vi "Store_single_subvi.vi"(3 "Parameter":u32(ring)=2049184 items=["SENSOR MODE"=4212128, "CCD MODE"=4212384, "READOUT MODE"=4211872, "ACTIVE VIEW INDEX"=4343136, "BITS PER CHANNEL"=4342976, "IMAGE PIXEL TYPE"=4343296, "BINNING"=4215968, "EXPOSURE TIME"=2049184, "CONTRAST GAIN"=3163312, "CONTRAST OFFSET"=3163328, "LIGHT MODE"=2114720, "SENSITIVITY"=2114992, "PHOTON IMAGING MODE"=2115200, "HIGH DYNAMIC RANGE MODE"=3163360, "WHITE BALANCE"=3163568, "TEMPERATURE"=2115232, "TEMPERATURE TARGET"=2115264, "SENSOR COOLER FAN"=2115296, "LINEBUNDLE HEIGHT"=4212192, "MECHANICAL SHUTTER"=2115488, "BACK FOCUS POSITION"=8422304, "TRIGGER CONNECTOR"=1066432, "TRIGGER SOURCE"=1066144, "OUTPUT TRIGGER SOURCE"=1852576, "TRIGGER GLOBAL EXPOSURE"=2049680, "FIRST TRIGGER BEHAVIOR"=2049696, "CHANNEL SYNC"=1852352, "READOUT DIRECTION"=4211904, "PRE HSYNC COUNT"=1852704, "INTERNAL LINE SPEED"=4226000, "INTERNAL LINE INTERVAL"=4226016], 4 "Set":dbl=0.5, 5 "Frames":i32=1, 6 "File":path=path "D:/test", 7 "save":bool=TRUE caption="Blank Button") -> (0 "Display":T1(plugin-control), 1 "DCAM Version":string, 2 "Library Version":string)   [LabVIEW 2016]
uses:
  Global_Variates.vi
panel:
  in  "w2 2":i32
  in  "w1 2":i32
  in  "h2 2":i32
  in  "h1 2":i32
  in  "w2":i32=2048 min=0 max=2048 step=1
  in  "w1":i32 min=0 max=2048 step=1
  in  "h2":i32=2048 min=0 max=2048 step=1
  in  "h1":i32 min=0 max=2048 step=1
  out "w2-1":dbl format="%#_13g"
  out "h2-1":dbl format="%#_13g"
  # "中间亮斑"
  # "裁剪图片"
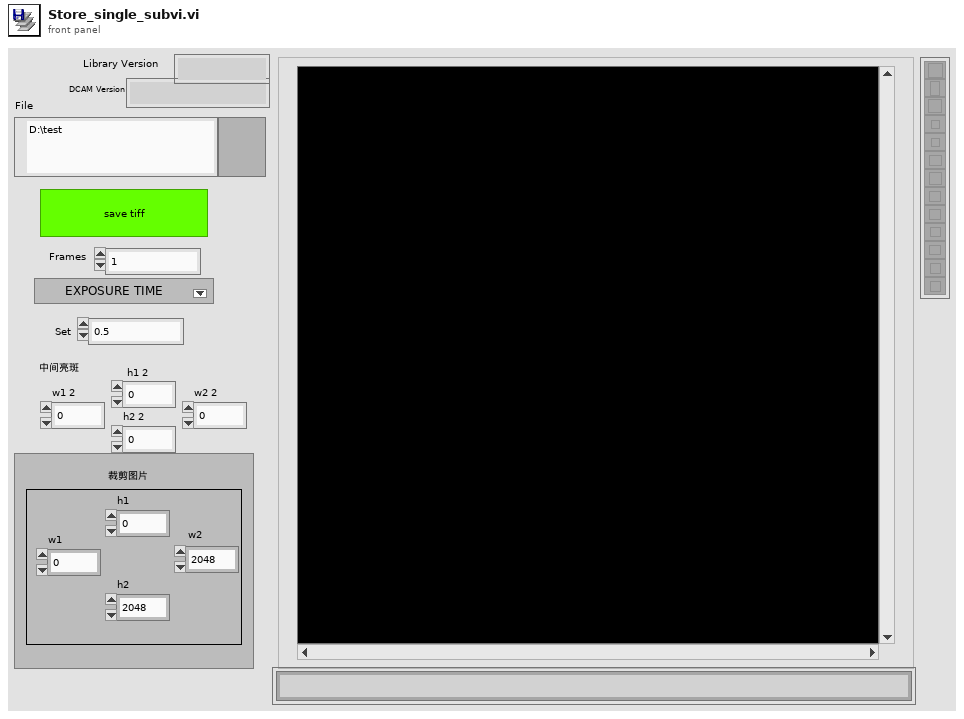
[diagram p1: front panel]
types:
  T1 = typedef "IMAQ Image.ctl" = refnum<image>
  T2 = cluster{"Capture Library":string, "DCAM-API":string}
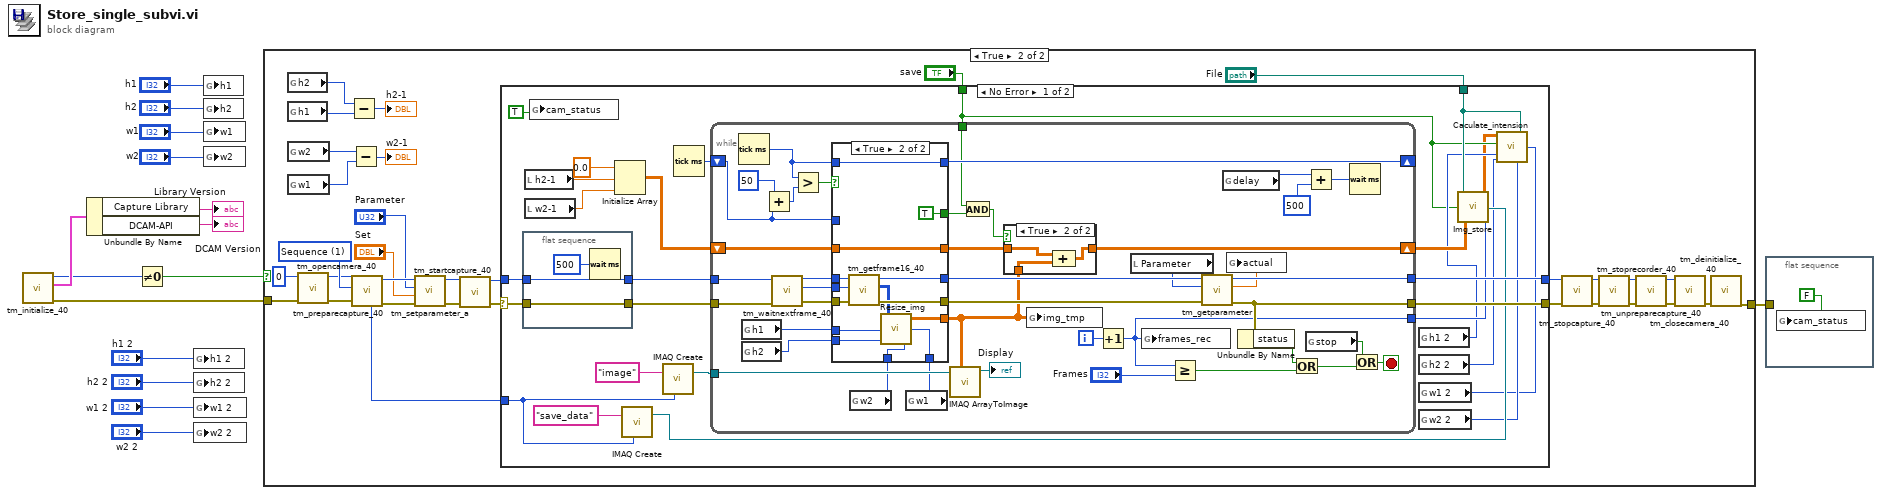
[diagram p0: block diagram]
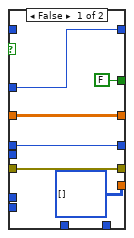
[diagram p4: hidden frame]
diagram:
  n1 = call <userlib>:"tm_initialize_40.vi"() -> ("error out"=w14:errorcluster, "Version Info"=w11:T2, "Number Of Cameras"=w10:u32)  [unwired: 8 in, 1 out]
  n2 = Unbundle By Name(w11) -> ("Capture Library"=→"Library Version":string, "DCAM-API"=→"DCAM Version":string)
  n3 = Not Equal To 0?(x=w10) -> (x != 0?=w9:bool)
  n4 = global write "Global_Variates.vi" "h1 2"("h1 2") -> ()
  n5 = global write "Global_Variates.vi" "h2 2"("h2 2") -> ()
  n6 = global write "Global_Variates.vi" "w1 2"("w1 2") -> ()
  n7 = global write "Global_Variates.vi" "w2 2"("w2 2") -> ()
  n8 = global write "Global_Variates.vi" "h1"("h1") -> ()
  n9 = global write "Global_Variates.vi" "h2"("h2") -> ()
  n10 = global write "Global_Variates.vi" "w1"("w1") -> ()
  n11 = global write "Global_Variates.vi" "w2"("w2") -> ()
  n12 = case shown="True" w9 {
    tunnel: w14 -> [w16 w48]
    tunnel: [w16 w31] -> w15
    frame False {
    }
    frame True {
      w43 = 1 items=["Snap", "Sequence"] ("Capture mode")
      n13 = global read "Global_Variates.vi" "h2"() -> (w22:i32)
      n14 = global read "Global_Variates.vi" "h1"() -> (w21:i32)
      n15 = global read "Global_Variates.vi" "w2"() -> (w18:i32)
      n16 = global read "Global_Variates.vi" "w1"() -> (w17:i32)
      n17 = call <userlib>:"tm_opencamera_40.vi"("error in (no error)"=w48, "Camera Index"=u32 0) -> ("error out"=w41:errorcluster, "Handle out"=w42:u32)  [unwired: 7 in, 1 out]
      n18 = Subtract(x=w22, y=w21) -> (x-y=→"h2-1":i32)
      n19 = Subtract(x=w18, y=w17) -> (x-y=→"w2-1":i32)
      n20 = call <userlib>:"tm_preparecapture_40.vi"("error in (no error)"=w41, "Capture mode"=w43, "Handle in"=w42) -> ("error out"=w33:errorcluster, "Handle out"=w34:u32, "Image type"=w29:u32)  [unwired: 5 in, 1 out]
      n21 = call <userlib>:"tm_setparameter_a.vi"("error in (no error)"=w33, "Value in"="Set", "Parameter"="Parameter", "Handle in"=w34) -> ("error out"=w27:errorcluster, "Handle out"=w28:u32)  [unwired: 6 in]
      n22 = call <userlib>:"tm_startcapture_40.vi"("error in (no error)"=w27, "Handle in"=w28) -> ("error out"=w35:errorcluster, "Handle out"=w24:u32)  [unwired: 8 in]
      n23 = case shown="No Error" w35 {
        selector: w35 -> [w67 w143]
        tunnel: w24 -> [w71 w144]
        tunnel: [w73 w144] -> w37
        tunnel: [w72 w143] -> w36
        tunnel: w29 -> [w64 _]
        tunnel: "save" -> [w50 _]
        tunnel: "File" -> [w55 _]
        frame No Error {
          n24 = flat-sequence {
            tunnel: w71 -> [w77]
            tunnel: [w77] -> w70
            tunnel: w67 -> [w75]
            tunnel: [w75] -> w66
            frame #0 {
              n25 = Wait (ms)(milliseconds to wait=u32 500) -> ()  [unwired: 1 out]
            }
          }
          n26 = local read "h2-1"() -> (w59:dbl)
          n27 = local read "w2-1"() -> (w58:dbl)
          n28 = global write "Global_Variates.vi" "cam_status"(TRUE) -> ()
          n29 = Initialize Array(0.0 ("element"), w59, w58) -> (w57:dbl[][])
          n30 = call "IMAQ Create"("Image Name"="save_data", "Image Type"=w64) -> ("New Image"=w61:T1)  [unwired: 3 in, 1 out]
          n31 = call "IMAQ Create"("Image Name"="image", "Image Type"=w64) -> ("New Image"=w62:T1)  [unwired: 3 in, 1 out]
          n32 = Tick Count (ms)() -> (millisecond timer value=w74:u32)
          n33 = while {
            tunnel: [w108] -> w73
            tunnel: [w107] -> w72
            tunnel: w70 -> [w117]
            tunnel: w66 -> [w118]
            shift-right: [w110] -> _
            shift-left: w74 -> [w91]
            shift-right: [w96] -> w56
            shift-left: w57 -> [w101]
            tunnel: w62 -> [w99]
            tunnel: w50 -> [w90]
            tunnel: [w87] -> w63
            i -> [w102]
            stop <- w104 stop-if-true
            n34 = Tick Count (ms)() -> (millisecond timer value=w111:u32)
            n35 = global read "Global_Variates.vi" "h1"() -> (w85:i32)
            n36 = global read "Global_Variates.vi" "h2"() -> (w84:i32)
            n37 = Add(x=u32 50, y=w91) -> (x+y=w112:u32)
            n38 = call <userlib>:"tm_waitnextframe_40.vi"("error in (no error)"=w118, "Handle in"=w117) -> ("error out"=w115:errorcluster, "Frame Index"=w114:i32, "Handle out"=w116:u32)  [unwired: 6 in, 1 out]
            n39 = Greater?(x=w111, y=w112) -> (0:w98:bool)
            n40 = global read "Global_Variates.vi" "w2"() -> (w83:i32)
            n41 = global read "Global_Variates.vi" "w1"() -> (w82:i32)
            n42 = case shown="True" w98 {
              tunnel: w116 -> [w125 w142]
              tunnel: w115 -> [w126 w140]
              tunnel: w114 -> [_ w141]
              tunnel: w91 -> [w128 _]
              tunnel: w111 -> [_ w137]
              tunnel: [w125 w138] -> w109
              tunnel: [w128 w137] -> w110
              tunnel: [w126 w139] -> w103
              tunnel: [w127 w136] -> w97
              tunnel: w101 -> [w127 w136]
              tunnel: [u16[][] [] ("Data") w133] -> w78
              tunnel: [FALSE TRUE] -> w88
              tunnel: w85 -> [_ w132]
              tunnel: w84 -> [_ w131]
              tunnel: w82 -> [_ w130]
              tunnel: w83 -> [_ w129]
              frame False {
              }
              frame True {
                n43 = call <userlib>:"tm_getframe16_40.vi"("error in (no error)"=w140, "Frame Index"=w141, "Handle in"=w142) -> ("error out"=w139:errorcluster, "Data"=w134:u16[][], "Handle out"=w138:u32)  [unwired: 5 in, 1 out]
                n44 = call "Resize_img.vi"("w2"=w129, "w1"=w130, "h2"=w131, "h1"=w132, "img_in"=w134) -> ("img_out"=w133:dbl[][])
              }
            }
            n45 = call "IMAQ ArrayToImage"("Image Pixels (U16)"=w78, "Image"=w99) -> ("Image Out"=→"Display":T1)  [unwired: 8 in, 1 out]
            n46 = And(x=w90, y=w88) -> (x .and. y?=w89:bool)
            n47 = case shown="True" w89 {
              tunnel: w97 -> [w119 w122]
              tunnel: [w119 w121] -> w96
              tunnel: w78 -> [_ w120]
              frame False {
              }
              frame True {
                n48 = Compound Arithmetic op=ADD(w122, w120) -> (w121:dbl[][])
              }
            }
            n49 = global write "Global_Variates.vi" "img_tmp"(w78) -> ()
            n50 = Increment(x=w102) -> (x+1=w87:i32)
            n51 = local read "Parameter"() -> (w94:u32)
            n52 = global write "Global_Variates.vi" "frames_rec"(w87) -> ()
            n53 = Greater Or Equal?(x=w87, y="Frames") -> (x >= y?=w105:bool)
            n54 = call <userlib>:"tm_getparameter.vi"("error in (no error)"=w103, "Parameter"=w94, "Handle in"=w109) -> ("error out"=w107:errorcluster, "Value out"=w95:dbl, "Handle out"=w108:u32)  [unwired: 6 in]
            n55 = global read "Global_Variates.vi" "delay"() -> (w79:i32)
            n56 = global write "Global_Variates.vi" "actual"(w95) -> ()
            n57 = Unbundle By Name(w107) -> ("status"=w106:bool)
            n58 = Or(x=w106, y=w105) -> (x .or. y?=w93:bool)
            n59 = Add(x=w79, y=u32 500 ("milliseconds to wait")) -> (x+y=w80:u32)
            n60 = global read "Global_Variates.vi" "stop"() -> (w92:bool)
            n61 = Wait (ms)(milliseconds to wait=w80) -> ()  [unwired: 1 out]
            n62 = Or(x=w92, y=w93) -> (x .or. y?=w104:bool)
          }
          n63 = global read "Global_Variates.vi" "h1 2"() -> (w51:i32)
          n64 = global read "Global_Variates.vi" "h2 2"() -> (w52:i32)
          n65 = global read "Global_Variates.vi" "w1 2"() -> (w53:i32)
          n66 = global read "Global_Variates.vi" "w2 2"() -> (w54:i32)
          n67 = call "Img_store.vi"("total"=w63, "img_in"=w61, "img_data"=w56, "save"=w50, "Path"=w55) -> ("img_one"=w49:dbl[][])
          n68 = call "Caculate_intension.vi"("w2"=w54, "w1"=w53, "file path"=w55, "h2"=w52, "h1"=w51, "Boolean"=w50, "img_data"=w49) -> ()
        }
        frame Error {
        }
      }
      n69 = call <userlib>:"tm_stopcapture_40.vi"("error in (no error)"=w36, "Handle in"=w37) -> ("error out"=w30:errorcluster, "Handle out"=w40:u32)  [unwired: 8 in]
      n70 = call <userlib>:"tm_stoprecorder_40.vi"("error in (no error)"=w30, "Handle in"=w40) -> ("error out"=w38:errorcluster, "Handle out"=w39:u32)  [unwired: 8 in]
      n71 = call <userlib>:"tm_unpreparecapture_40.vi"("error in (no error)"=w38, "Handle in"=w39) -> ("error out"=w45:errorcluster, "Handle out"=w44:u32)  [unwired: 8 in]
      n72 = call <userlib>:"tm_closecamera_40.vi"("error in (no error)"=w45, "Handle in"=w44) -> ("error out"=w46:errorcluster)  [unwired: 9 in]
      n73 = call <userlib>:"tm_deinitialize_40.vi"("error in (no error)"=w46) -> ("error out"=w31:errorcluster)  [unwired: 10 in]
    }
  }
  n74 = flat-sequence {
    tunnel: w15 -> [_]
    frame #0 {
      n75 = global write "Global_Variates.vi" "cam_status"(FALSE) -> ()
    }
  }
